vi "CRYSet Calibration Front Panel.vi"(11 "Vi Ref":refnum<vi>) -> ()   [LabVIEW 2013]
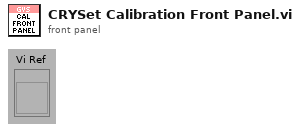
[diagram p1: front panel]
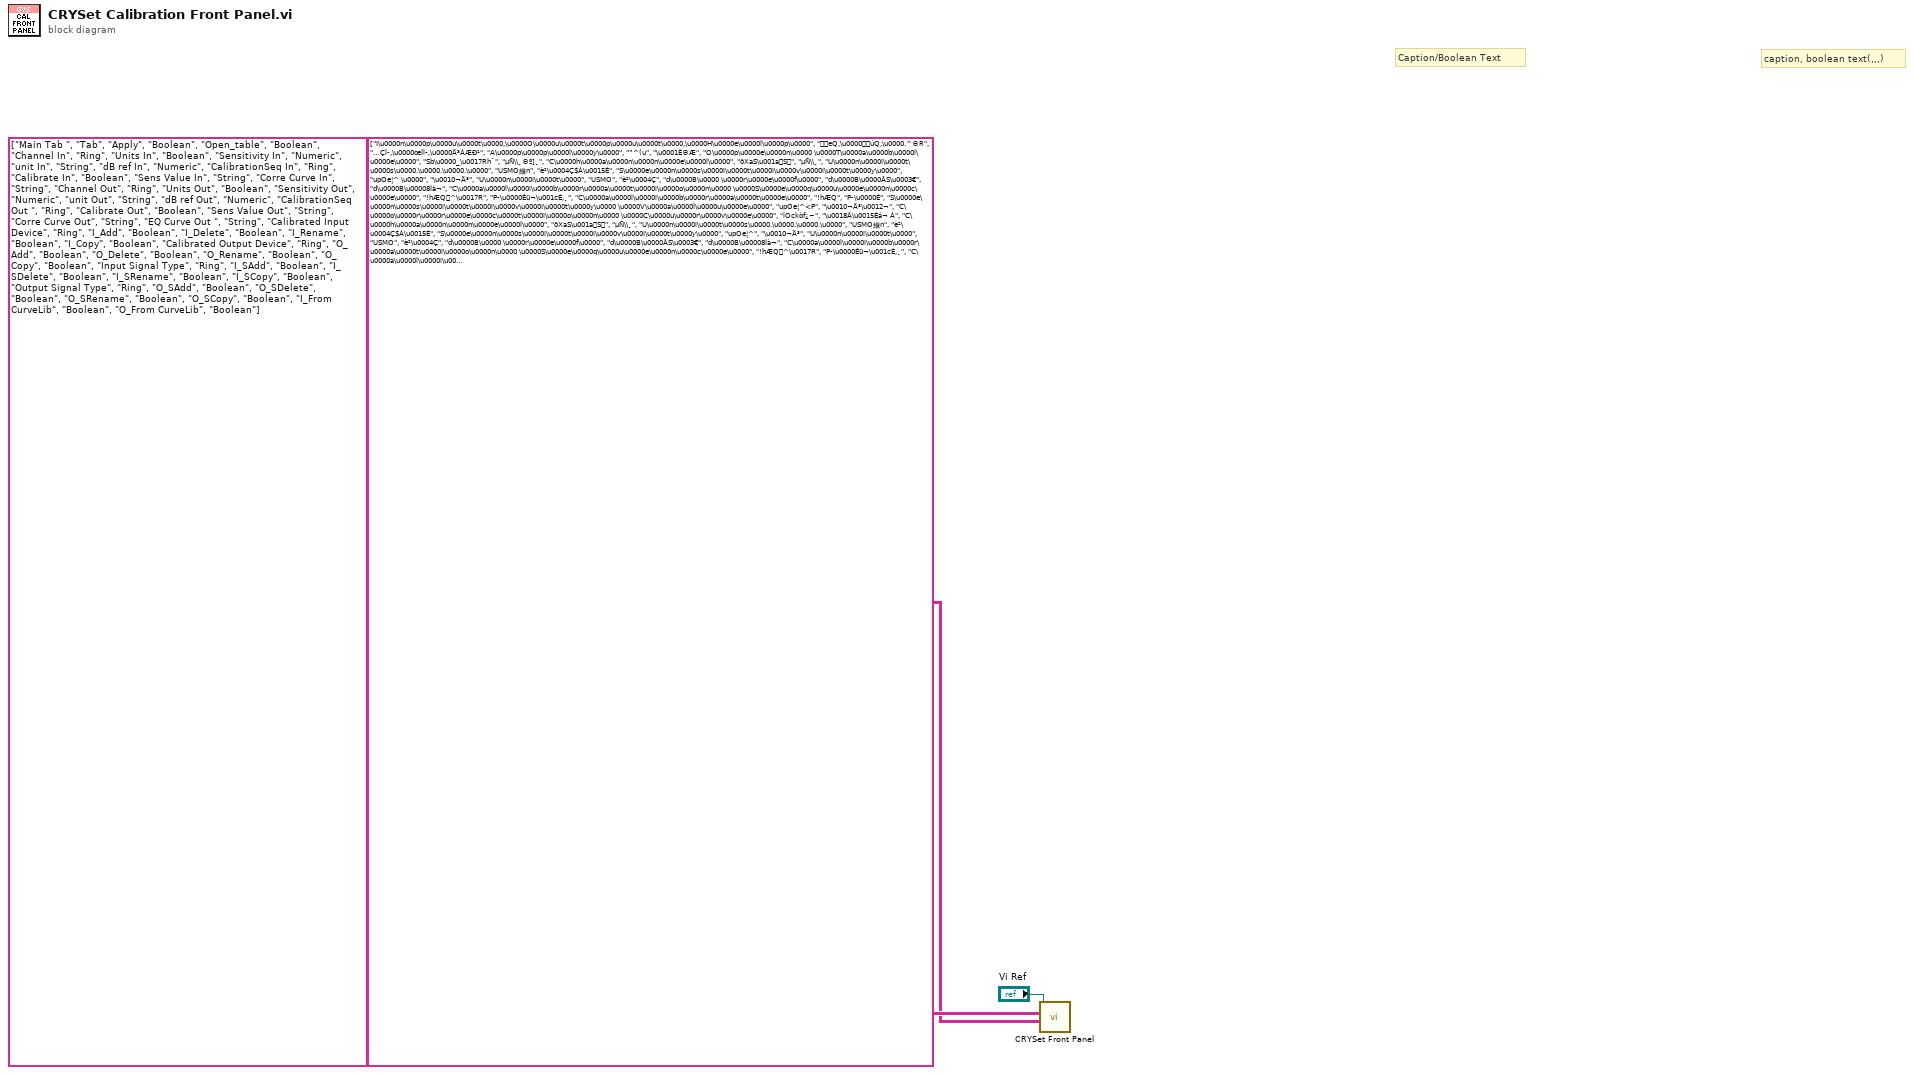
[diagram p0: block diagram]
diagram:
  # "Caption, Tab Page, Multilist Header, Button 4"
  # "Control Type"
  # "Control Name and Tab"
  # "caption, boolean text(,,,)"
  # "Caption/Boolean Text"
  n1 = call "CRYSet Front Panel.vi"("Caption(Boolean Text)"=string[][] [["I\u0000n\u0000p\u0000u\u0000t\u0000,\u0000O\u0000u\u0000t\u0000p\u0000u\u0000t\u0000,\u0000H\u0000e\u0000l\u0000p\u0000", "eQ,\u0000úQ,\u0000.^©R", "…Çl­,\u0000œÍl­,\u0000Ä³ÀÆÐ¹"], ["A\u0000p\u0000p\u0000l\u0000y\u0000", "”^(u", "\u0001È©Æ"], ["O\u0000p\u0000e\u0000n\u0000 \u0000T\u0000a\u0000b\u0000l\u0000e\u0000", "Sb\u0000_\u0017Rhˆ", "µÑ\\¸©º]¸"], ["C\u0000h\u0000a\u0000n\u0000n\u0000e\u0000l\u0000", "ðXaS\u001aS", "µÑ\\¸"], ["U\u0000n\u0000i\u0000t\u0000s\u0000.\u0000.\u0000.\u0000", "USMO緥n", "è²\u0004Ç$Á\u0015È"], ["S\u0000e\u0000n\u0000s\u0000i\u0000t\u0000i\u0000v\u0000i\u0000t\u0000y\u0000", "upOe¦^ \u0000", "\u0010¬Ä³"], ["U\u0000n\u0000i\u0000t\u0000", "USMO", "è²\u0004Ç"], ["d\u0000B\u0000 \u0000r\u0000e\u0000f\u0000", "d\u0000B\u0000ÂS\u0003€", "d\u0000B\u00008Ìà¬"], ["C\u0000a\u0000l\u0000i\u0000b\u0000r\u0000a\u0000t\u0000i\u0000o\u0000n\u0000 \u0000S\u0000e\u0000q\u0000u\u0000e\u0000n\u0000c\u0000e\u0000", "!hÆQ^\u0017R", "P­\u0000Éü¬\u001cÈ,¸"], ["C\u0000a\u0000l\u0000i\u0000b\u0000r\u0000a\u0000t\u0000e\u0000", "!hÆQ", "P­\u0000É"], ["S\u0000e\u0000n\u0000s\u0000i\u0000t\u0000i\u0000v\u0000i\u0000t\u0000y\u0000 \u0000V\u0000a\u0000l\u0000u\u0000e\u0000", "upOe¦^<P", "\u0010¬Ä³\u0012¬"], ["C\u0000o\u0000r\u0000r\u0000e\u0000c\u0000t\u0000i\u0000o\u0000n\u0000 \u0000C\u0000u\u0000r\u0000v\u0000e\u0000", "îOckòf¿~", "\u0018Â\u0015Èá¬ Á"], ["C\u0000h\u0000a\u0000n\u0000n\u0000e\u0000l\u0000", "ðXaS\u001aS", "µÑ\\¸"], ["U\u0000n\u0000i\u0000t\u0000s\u0000.\u0000.\u0000.\u0000", "USMO緥n", "è²\u0004Ç$Á\u0015È"], ["S\u0000e\u0000n\u0000s\u0000i\u0000t\u0000i\u0000v\u0000i\u0000t\u0000y\u0000", "upOe¦^", "\u0010¬Ä³"], ["U\u0000n\u0000i\u0000t\u0000", "USMO", "è²\u0004Ç"], ["d\u0000B\u0000 \u0000r\u0000e\u0000f\u0000", "d\u0000B\u0000ÂS\u0003€", "d\u0000B\u00008Ìà¬"], ["C\u0000a\u0000l\u0000i\u0000b\u0000r\u0000a\u0000t\u0000i\u0000o\u0000n\u0000 \u0000S\u0000e\u0000q\u0000u\u0000e\u0000n\u0000c\u0000e\u0000", "!hÆQ^\u0017R", "P­\u0000Éü¬\u001cÈ,¸"], ["C\u0000a\u0000l\u0000i\u0000b\u0000r\u0000a\u0000t\u0000e\u0000", "!hÆQ", "P­\u0000É"], ["S\u0000e\u0000n\u0000s\u0000i\u0000t\u0000i\u0000v\u0000i\u0000t\u0000y\u0000 \u0000V\u0000a\u0000l\u0000u\u0000e\u0000", "upOe¦^<P", "\u0010¬Ä³\u0012¬"], ["C\u0000o\u0000r\u0000r\u0000e\u0000c\u0000t\u0000i\u0000o\u0000n\u0000 \u0000C\u0000u\u0000r\u0000v\u0000e\u0000", "îOckòf¿~", "\u0018Â\u0015Èá¬ Á"], ["E\u0000Q\u0000 \u0000C\u0000u\u0000r\u0000v\u0000e\u0000", "GWaˆhVòf¿~", "à­ñ´TÖá¬ Á"], ["C\u0000a\u0000l\u0000i\u0000b\u0000r\u0000a\u0000t\u0000e\u0000d\u0000 \u0000I\u0000n\u0000p\u0000u\u0000t\u0000 \u0000D\u0000e\u0000v\u0000i\u0000c\u0000e\u0000", "!hÆQeQ¾\u0007Y", "P­\u0000É\\Õ \u0000…Çl­¥ÇXÎ"], ["A\u0000d\u0000d\u0000", "ûm R", "”Í\u0000¬"], ["D\u0000e\u0000l\u0000e\u0000t\u0000e\u0000", " Rd–", "­À\u001cÈ"], ["R\u0000e\u0000n\u0000a\u0000m\u0000e\u0000", "͑}T\rT", "兰浆"], ["C\u0000o\u0000p\u0000y\u0000", "\rY6R", "õ¼¬À"], ["C\u0000a\u0000l\u0000i\u0000b\u0000r\u0000a\u0000t\u0000e\u0000d\u0000 \u0000O\u0000u\u0000t\u0000p\u0000u\u0000t\u0000 \u0000D\u0000e\u0000v\u0000i\u0000c\u0000e\u0000", "!hÆQúQ¾\u0007Y", "P­\u0000É\\Õ \u0000œÍl­¥ÇXÎ"], ["A\u0000d\u0000d\u0000", "ûm R", "”Í\u0000¬"], ["D\u0000e\u0000l\u0000e\u0000t\u0000e\u0000", " Rd–", "­À\u001cÈ"], ["R\u0000e\u0000n\u0000a\u0000m\u0000e\u0000", "͑}T\rT", "兰浆"], ["C\u0000o\u0000p\u0000y\u0000", "\rY6R", "õ¼¬À"], ["I\u0000n\u0000p\u0000u\u0000t\u0000 \u0000S\u0000i\u0000g\u0000n\u0000a\u0000l\u0000 \u0000T\u0000y\u0000p\u0000e\u0000", "eQáO÷S\u001aS", "…Çl­àÂ8Ö\u0015ÖÜÐ"], ["A\u0000d\u0000d\u0000", "ûm R", "”Í\u0000¬"], ["D\u0000e\u0000l\u0000e\u0000t\u0000e\u0000", " Rd–", "­À\u001cÈ"], ["R\u0000e\u0000n\u0000a\u0000m\u0000e\u0000", "͑}T\rT", "兰浆"], ["C\u0000o\u0000p\u0000y\u0000", "\rY6R", "õ¼¬À"], ["O\u0000u\u0000t\u0000p\u0000u\u0000t\u0000 \u0000S\u0000i\u0000g\u0000n\u0000a\u0000l\u0000 \u0000T\u0000y\u0000p\u0000e\u0000", "úQáO÷S\u001aS", "œÍl­àÂ8Ö\u0015ÖÜÐ"], ["A\u0000d\u0000d\u0000", "ûm R", "”Í\u0000¬"], ["D\u0000e\u0000l\u0000e\u0000t\u0000e\u0000", " Rd–", "­À\u001cÈ"], ["R\u0000e\u0000n\u0000a\u0000m\u0000e\u0000", "͑}T\rT", "兰浆"], ["C\u0000o\u0000p\u0000y\u0000", "\rY6R", "õ¼¬À"], ["C\u0000o\u0000p\u0000y\u0000 \u0000F\u0000r\u0000o\u0000m\u0000 \u0000C\u0000u\u0000r\u0000v\u0000e\u0000 \u0000L\u0000i\u0000b\u0000r\u0000a\u0000r\u0000y\u0000", "ÎNòf¿~“^\rY6R", "á¬ Á\u001cÁà¬ÐÅ\u001cÁ \u0000õ¼¬À"], ["C\u0000o\u0000p\u0000y\u0000 \u0000F\u0000r\u0000o\u0000m\u0000 \u0000C\u0000u\u0000r\u0000v\u0000e\u0000 \u0000L\u0000i\u0000b\u0000r\u0000a\u0000r\u0000y\u0000", "ÎNòf¿~“^\rY6R", "á¬ Á\u001cÁà¬ÐÅ\u001cÁ \u0000õ¼¬À"]], "Control ID and Type(Label Name, Type)"=string[][] [["Main Tab ", "Tab"], ["Apply", "Boolean"], ["Open_table", "Boolean"], ["Channel In", "Ring"], ["Units In", "Boolean"], ["Sensitivity In", "Numeric"], ["unit In", "String"], ["dB ref In", "Numeric"], ["CalibrationSeq In", "Ring"], ["Calibrate In", "Boolean"], ["Sens Value In", "String"], ["Corre Curve In", "String"], ["Channel Out", "Ring"], ["Units Out", "Boolean"], ["Sensitivity Out", "Numeric"], ["unit Out", "String"], ["dB ref Out", "Numeric"], ["CalibrationSeq Out ", "Ring"], ["Calibrate Out", "Boolean"], ["Sens Value Out", "String"], ["Corre Curve Out", "String"], ["EQ Curve Out ", "String"], ["Calibrated Input Device", "Ring"], ["I_Add", "Boolean"], ["I_Delete", "Boolean"], ["I_Rename", "Boolean"], ["I_Copy", "Boolean"], ["Calibrated Output Device", "Ring"], ["O_Add", "Boolean"], ["O_Delete", "Boolean"], ["O_Rename", "Boolean"], ["O_Copy", "Boolean"], ["Input Signal Type", "Ring"], ["I_SAdd", "Boolean"], ["I_SDelete", "Boolean"], ["I_SRename", "Boolean"], ["I_SCopy", "Boolean"], ["Output Signal Type", "Ring"], ["O_SAdd", "Boolean"], ["O_SDelete", "Boolean"], ["O_SRename", "Boolean"], ["O_SCopy", "Boolean"], ["I_From CurveLib", "Boolean"], ["O_From CurveLib", "Boolean"]], "Vi Ref"="Vi Ref") -> ()  [unwired: 9 in]
